vi "OCV Send GUN Trigger.vi"(8 "error in (no error)":errorcluster, 11 "Refnum in":refnum<k21>) -> (0 "error out":errorcluster, 3 "Refnum out":refnum<k21>, 4 "Gun Trig Time":u32)   [LabVIEW 2019]
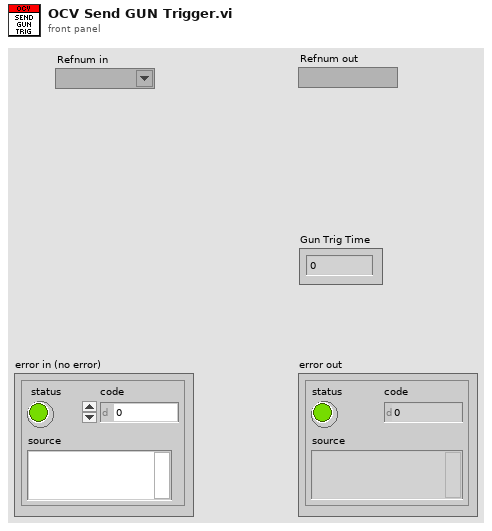
[diagram p1: front panel]
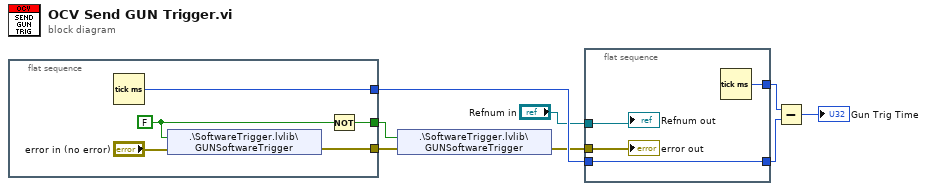
[diagram p0: block diagram]
diagram:
  n1 = flat-sequence {
    tunnel: [w12] -> w8
    tunnel: [w10] -> w4
    tunnel: [w9] -> w3
    frame #0 {
      w11 = FALSE ("GUNSoftwareTrigger")
      n2 = Tick Count (ms)() -> (millisecond timer value=w12:u32)
      n3 = shared-variable ".\\SoftwareTrigger.lvlib\\GUNSoftwareTrigger"(w11, error in="error in (no error)") -> (error out=w9:errorcluster)
      n4 = Not(x=w11) -> (.not. x?=w10:bool)
    }
  }
  n5 = shared-variable ".\\SoftwareTrigger.lvlib\\GUNSoftwareTrigger"(w4, error in=w3) -> (error out=w2:errorcluster)
  n6 = flat-sequence {
    tunnel: [w17] -> w7
    tunnel: "Refnum in" -> [w15]
    tunnel: w2 -> [w16]
    tunnel: w8 -> [w14]
    tunnel: [w14] -> w6
    frame #0 {
      n7 = Tick Count (ms)() -> (millisecond timer value=w17:u32)
      "Refnum out" <- w15
      "error out" <- w16
    }
  }
  n8 = Subtract(x=w7, y=w6) -> (x-y=→"Gun Trig Time":u32)
